vi "FRCts20_Backend_Stats_GET.vi"(6 "Message Attributes":T4, 8 "error in (no error)":errorcluster, 10 "Data":string, 11 "Engine_Refnums":T1) -> (0 "error out":errorcluster)   [LabVIEW 2014, in "FRCts20_Backend_Engine.lvlib"]
doc: "Returns all statistics for a given competition. Called by the stats API. Expects competition name. Takes many ms to complete, as it involves multiple calls to the database. This is somewhat mitigated by the large amount of parallelism in the VI, but even a basic db takes 7-12 ms to return statistics."
uses:
  FRCts20_Backend_Engine.lvlib
  Dependencies/Keyed Array/KeyedArray.ctl
  FRCts20_Backend_EngineRefnums.ctl
  INI_Accessor/FRCts20_Backend_INI Controller.lvclass
  Dependencies/AMC/_SubVIs/TypeDefs/Message Queue.ctl
  Dependencies/AMC/_SubVIs/TypeDefs/Message.ctl
  <vilib>/addons/database/Connection.llb/Conn ObjectReference.ctl
  FRCts20_Backend_FGVOperation.ctl
  Dependencies/Keyed Array/Tools_KeyedArray.lvlib
  Dependencies/AMC/AMC.lvlib
  <vilib>/addons/database/NI_Database_API.lvlib
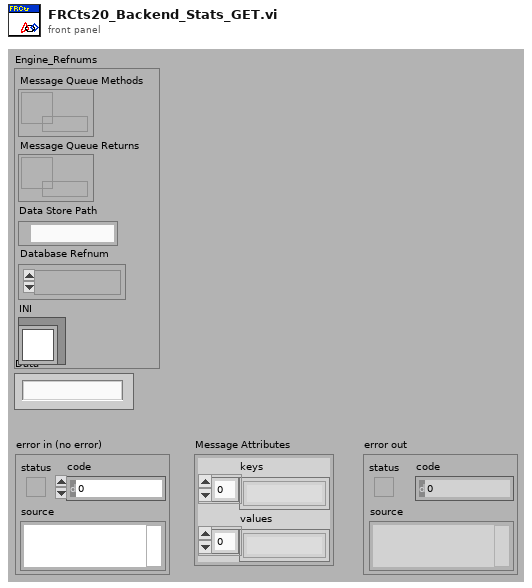
[diagram p1: front panel]
types:
  T1 = typedef "FRCts20_Backend_Engine.lvlib/FRCts20_Backend_EngineRefnums.ctl" = cluster{"Message Queue Methods":T2, "Message Queue Returns":T2, "Data Store Path":path, "Database Refnum":T3, "INI":refnum<class "FRCts20_Backend_INI Controller.lvclass">}
  T2 = typedef "AMC.lvlib/Message Queue.ctl" = refnum<queue>
  T3 = typedef "NI_Database_API.lvlib/Conn ObjectReference.ctl" = refnum<k1>
  T4 = typedef "Tools_KeyedArray.lvlib/KeyedArray.ctl" = cluster{"keys":string[], "values":string[]}
  T5 = typedef "FRCts20_Backend_Engine.lvlib/FRCts20_Backend_FGVOperation.ctl" = enum16{"Initialize", "EnqueueMessage", "EnqueueDataReturn", "FlushMessage", "FlushDataReturn"}
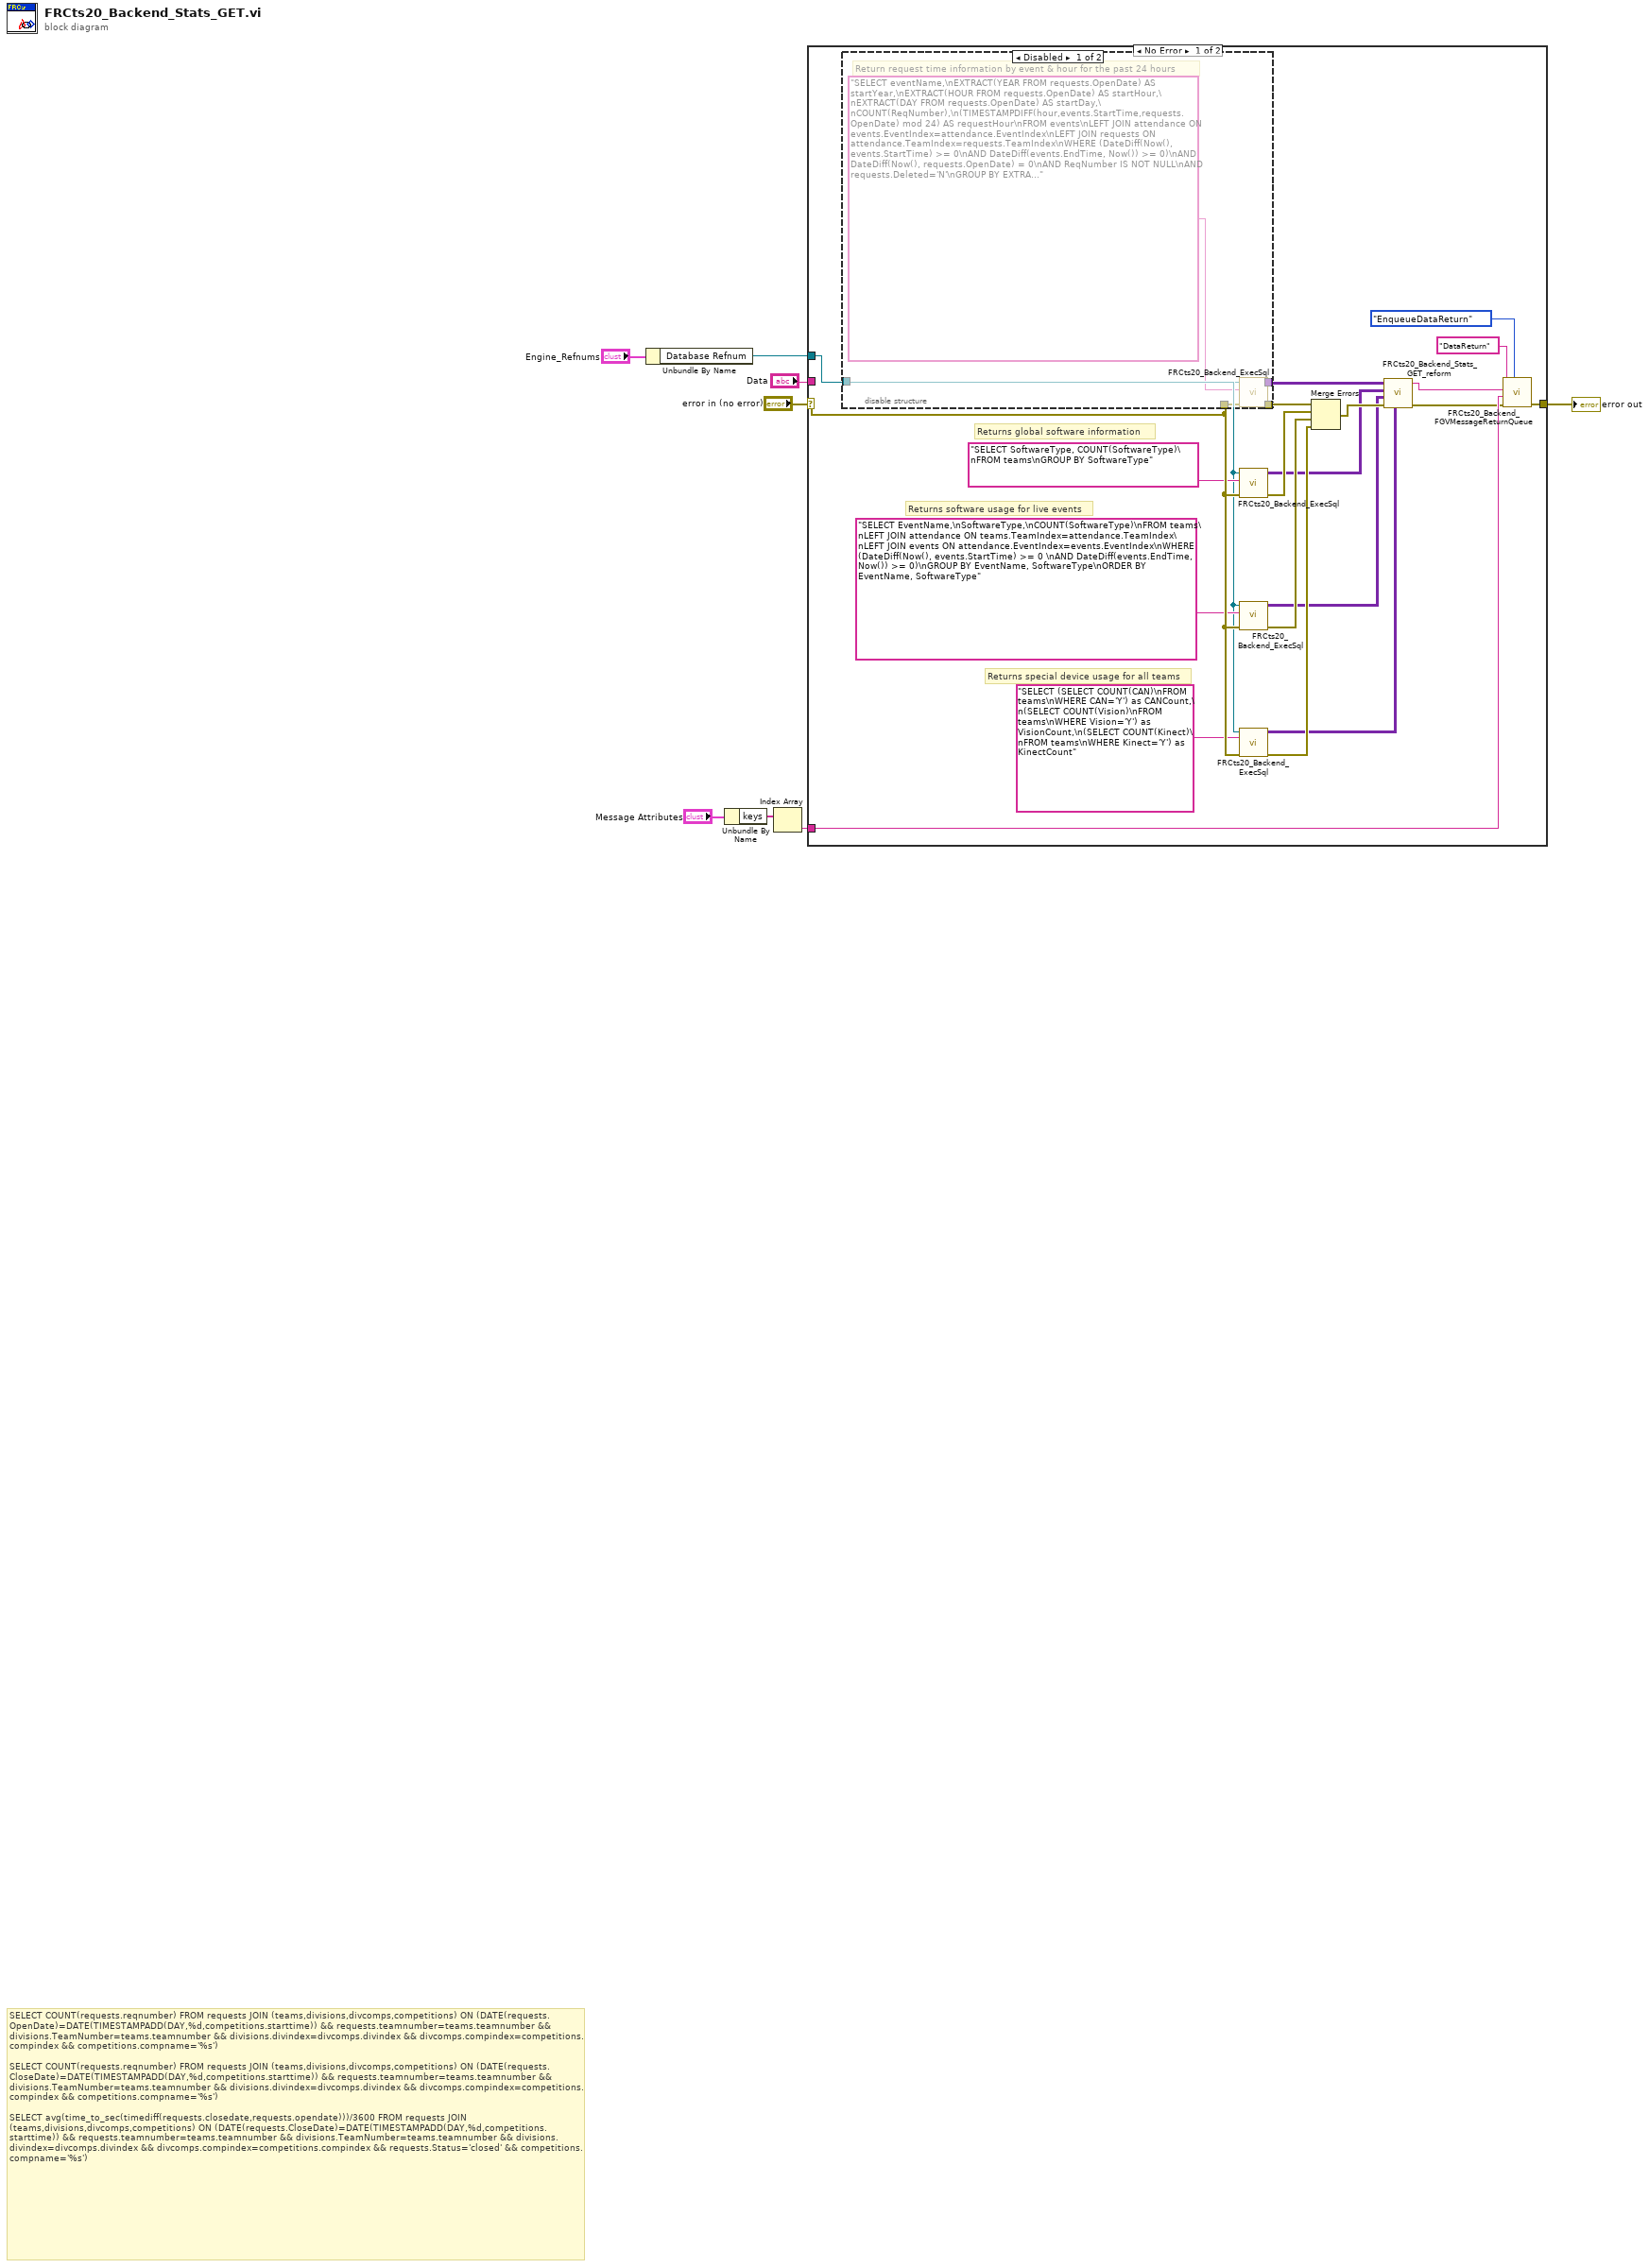
[diagram p0: block diagram]
diagram:
  # "SELECT COUNT(requests.reqnumber) FROM requests JOIN (teams,divisions,divcomps,competitions) ON (DATE(requests.OpenDate)=DATE(TIMESTAMPADD(DAY,%d,competitions.starttime)) && requests.teamnumber=teams.teamnumber && divisions.TeamNumber=teams.teamnumber && divisions.divindex=divcomps.divindex && divcomps.compindex=competitions.compindex && competitions.compname='%s')\n\nSELECT COUNT(requests.reqnumber) FROM requests JOIN (teams,divisions,divcomps,competitions) ON (DATE(requests.CloseDate)=DATE(TIMESTAMPADD(DAY,%d,competitions.starttime)) && requests.teamnumber=teams.teamnumber && divisions.TeamNumber=teams.teamnumber && divisions.divindex=divcomps.divindex && divcomps.compindex=competitions.compindex && competitions.compname='%s')\n\nSELECT avg(time_to_sec(timediff(requests.closedate,requests.opendate)))/3600 FROM requests JOIN (teams,divisions,divcomps,competitions) ON (DATE(requests.CloseDate)=DATE(TIMESTAMPADD(DAY,%d,competitions.starttime)) && requests.teamnumber=teams.teamnumber && divisions.TeamNumber=teams.teamnumber && divisions.divindex=divcomps.divindex && divcomps.compindex=competitions.compindex && requests.Status='closed' && competitions.compname='%s')"
  n1 = Unbundle By Name("Engine_Refnums") -> ("Database Refnum"=w3:T3)
  n2 = Unbundle By Name("Message Attributes") -> ("keys"=w7:string[])
  n3 = Index Array(array=w7) -> (element=w1:string)  [unwired: 1 in]
  n4 = case shown="No Error" "error in (no error)" {
    selector: "error in (no error)" -> [w24 w34]
    tunnel: [w25 w34] -> w4
    tunnel: w3 -> [w20 _]
    tunnel: "Data" -> [_ _]
    tunnel: w1 -> [w26 _]
    frame No Error {
      # "Returns special device usage for all teams"
      # "Returns software usage for live events"
      # "Returns global software information"
      n5 = disable-structure shown="Disabled" {
        disable-tunnel: w24 -> [w33 _]
        disable-tunnel: w20 -> [w31 _]
        disable-tunnel: [w30 _] -> w19
        disable-tunnel: [w29 _] -> w14
        frame Disabled {
          # "Return request time information by event & hour for the past 24 hours"
          n6 = call "FRCts20_Backend_ExecSql.vi"("error in (no error)"=w33, "format string"="SELECT eventName,\nEXTRACT(YEAR FROM requests.OpenDate) AS startYear,\nEXTRACT(HOUR FROM requests.OpenDate) AS startHour,\nEXTRACT(DAY FROM requests.OpenDate) AS startDay,\nCOUNT(ReqNumber),\n(TIMESTAMPDIFF(hour,events.StartTime,requests.OpenDate) mod 24) AS requestHour\nFROM events\nLEFT JOIN attendance ON events.EventIndex=attendance.EventIndex\nLEFT JOIN requests ON attendance.TeamIndex=requests.TeamIndex\nWHERE (DateDiff(Now(), events.StartTime) >= 0\nAND DateDiff(events.EndTime, Now()) >= 0)\nAND DateDiff(Now(), requests.OpenDate) = 0\nAND ReqNumber IS NOT NULL\nAND requests.Deleted='N'\nGROUP BY EXTRACT(DAY_HOUR FROM requests.OpenDate), eventName\nORDER BY EXTRACT(DAY_HOUR FROM requests.OpenDate)", "Refnum in"=w31) -> ("error out"=w30:errorcluster, "recordset data"=w29:variant[][])  [unwired: 6 in, 1 out]
        }
        frame Enabled {
        }
      }
      n7 = call "FRCts20_Backend_ExecSql.vi"("error in (no error)"=w24, "format string"="SELECT SoftwareType, COUNT(SoftwareType)\nFROM teams\nGROUP BY SoftwareType", "Refnum in"=w20) -> ("error out"=w18:errorcluster, "recordset data"=w11:variant[][])  [unwired: 6 in, 1 out]
      n8 = call "FRCts20_Backend_ExecSql.vi"("error in (no error)"=w24, "format string"="SELECT EventName,\nSoftwareType,\nCOUNT(SoftwareType)\nFROM teams\nLEFT JOIN attendance ON teams.TeamIndex=attendance.TeamIndex\nLEFT JOIN events ON attendance.EventIndex=events.EventIndex\nWHERE (DateDiff(Now(), events.StartTime) >= 0 \nAND DateDiff(events.EndTime, Now()) >= 0)\nGROUP BY EventName, SoftwareType\nORDER BY EventName, SoftwareType", "Refnum in"=w20) -> ("error out"=w17:errorcluster, "recordset data"=w13:variant[][])  [unwired: 6 in, 1 out]
      n9 = call "FRCts20_Backend_ExecSql.vi"("error in (no error)"=w24, "format string"="SELECT (SELECT COUNT(CAN)\nFROM teams\nWHERE CAN='Y') as CANCount,\n(SELECT COUNT(Vision)\nFROM teams\nWHERE Vision='Y') as VisionCount,\n(SELECT COUNT(Kinect)\nFROM teams\nWHERE Kinect='Y') as KinectCount", "Refnum in"=w20) -> ("error out"=w16:errorcluster, "recordset data"=w12:variant[][])  [unwired: 6 in, 1 out]
      n10 = Merge Errors(w19, w18, w17, w16) -> (w15:errorcluster)
      n11 = call "FRCts20_Backend_Stats_GET_reform.vi"("Special Device Usage"=w12, "Error In"=w15, "SW usage - Live Events"=w13, "Global SW Info"=w11, "Requests Per Hour"=w14) -> ("Error Out"=w10:errorcluster, "data string"=w9:string)  [unwired: 5 in]
      n12 = call "FRCts20_Backend_FGVMessageReturnQueue.vi"("Operation"=FRCts20_Backend_FGVOperation."EnqueueDataReturn", "error in (no error)"=w10, "Key"=w26, "Message Value"=w9, "Message Name"="DataReturn") -> ("error out"=w25:errorcluster)  [unwired: 5 in, 1 out]
    }
    frame Error {
    }
  }
  "error out" <- w4
